vi "myRIO_BRig_RT_dataExp_Cue1Param_CueType_Switch.vi"() -> (2 "output_Cue1Param_CueType_Switch":i32)   [LabVIEW 2014]
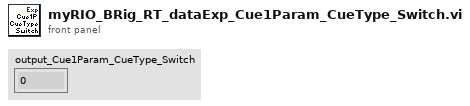
[diagram p1: front panel]
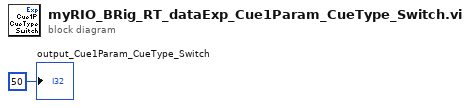
[diagram p0: block diagram]
diagram:
  "output_Cue1Param_CueType_Switch" <- 50 ("output_iBlock")
